vi "METIS_TestIOC_simple.vi"() -> ()   [LabVIEW 2020]
uses:
  2d31aa85-0ba4-4146-9dd6-b3e60546dde0.vi
  89720795-54a2-4534-9bbc-88a9e5af61a1.vi
  b2589dcb-5b22-4d43-a465-4351203ec25c.vi
  d910b247-ae28-4fff-85ad-f246d65b7ee6.vi
  f4696480-f13b-456b-91c7-c20ebdb2ee9c.vi
  <userlib>/caLab/Private/Put_I32-1D_PV-1D.vi
panel:
  in  "stop":bool
  in  "Min":i32=10
  in  "Bin":i32=5
  in  "X":i32=10
  in  "Y":i32=10
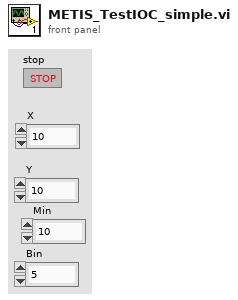
[diagram p1: front panel]
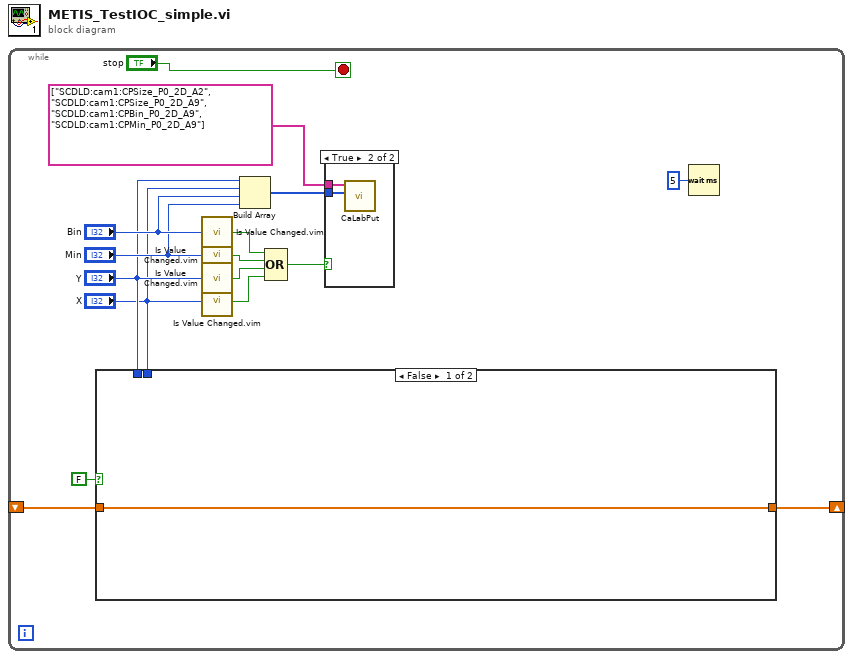
[diagram p0: block diagram]
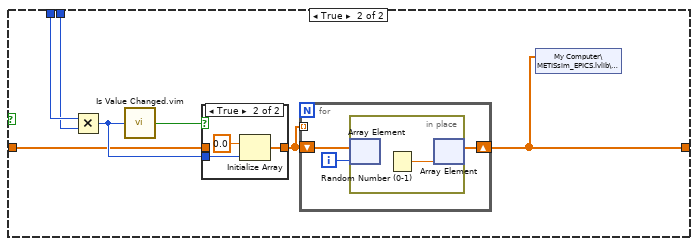
[diagram p2: hidden frame]
diagram:
  n1 = while {
    shift-right: [w3] -> _
    shift-left: _ -> [w4]
    stop <- "stop" stop-if-true
    n2 = case shown="False" FALSE {
      tunnel: "Y" -> [_ w24]
      tunnel: "X" -> [_ w23]
      tunnel: w4 -> [w17 w20]
      tunnel: [w17 w18] -> w3
      frame False {
      }
      frame True {
        n3 = Multiply(x=w24, y=w23) -> (x*y=w21:i32)
        n4 = call "Is Value Changed.vim"("value"=w21) -> ("changed or first call?"=w22:bool)
        n5 = case shown="True" w22 {
          tunnel: w21 -> [_ w31]
          tunnel: [w29 w30] -> w19
          tunnel: w20 -> [w29 _]
          frame False {
          }
          frame True {
            n6 = Initialize Array(0.0 ("element"), w31) -> (w30:dbl[])
          }
        }
        n7 = for {
          shift-right: [w25] -> w18
          shift-left: w19 -> [w27]
          tunnel: w19 -> [_] mode=indexing
          i -> [w26]
          n8 = in-place {
            n9 = in-place-array #1(w27, w26) -> ()  [unwired: 1 out]
            n10 = Random Number (0-1)() -> (number: 0 to 1=w28:dbl)
            n11 = in-place-array #1(w28) -> (w25:dbl[])  [unwired: 1 out]
          }
        }
        n12 = shared-variable "My Computer\\METISsim_EPICS.lvlib\\myData"(w18) -> ()  [unwired: 1 in, 1 out]
      }
    }
    n13 = call "Is Value Changed.vim"("value"="Bin") -> ("changed or first call?"=w11:bool)
    n14 = call "Is Value Changed.vim"("value"="Min") -> ("changed or first call?"=w10:bool)
    n15 = call "Is Value Changed.vim"("value"="Y") -> ("changed or first call?"=w15:bool)
    n16 = call "Is Value Changed.vim"("value"="X") -> ("changed or first call?"=w14:bool)
    n17 = Build Array("Y", "X", "Bin", "Min") -> (w8:i32[])
    n18 = Compound Arithmetic op=OR(w11, w10, w15, w14) -> (w9:bool)
    n19 = case shown="True" w9 {
      tunnel: w8 -> [_ w34]
      tunnel: string[] ["SCDLD:cam1:CPSize_P0_2D_A2", "SCDLD:cam1:CPSize_P0_2D_A9", "SCDLD:cam1:CPBin_P0_2D_A9", "SCDLD:cam1:CPMin_P0_2D_A9"] -> [_ w33]
      frame False {
      }
      frame True {
        n20 = call-poly <userlib>:"CaLabPut.vi"("Values"=w34, "PV Names"=w33) -> ()  [unwired: 6 in, 4 out]
      }
    }
    n21 = Wait (ms)(milliseconds to wait=u32 5) -> ()  [unwired: 1 out]
  }
